vi "Write Binary Config.vi"(4 "Include Class Name":bool, 6 "byte order (0:big-endian, network order)":T1(ring), 8 "error in (no error)":errorcluster, 11 "Const_WFM in":refnum<class "Const_WFM_1D.lvclass">) -> (0 "error out":errorcluster, 2 "Binary":string, 3 "Const_WFM out":refnum<class "Const_WFM_1D.lvclass">)   [LabVIEW 2021, in "Const_WFM_1D.lvclass"]
uses:
  Const_WFM_1D.lvclass
  Const_WFM_1D.lvclass/Const_WFM_1D.ctl
  Abs_Types/Waveform 1D/Abs_Waveform 1D.lvclass
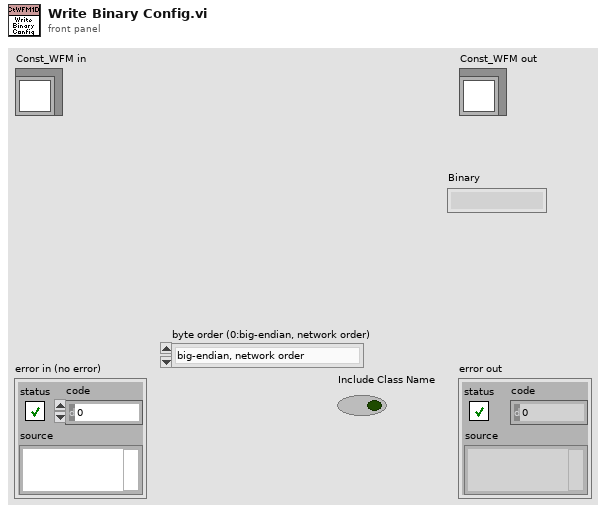
[diagram p1: front panel]
types:
  T1 = enum16{"big-endian, network order", "native, host order", "little-endian"}
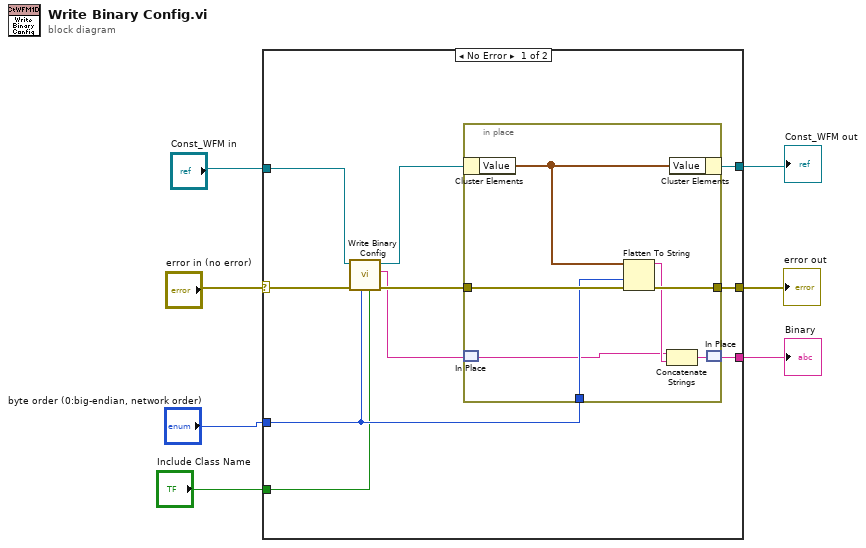
[diagram p0: block diagram]
diagram:
  n1 = case shown="No Error" "error in (no error)" {
    selector: "error in (no error)" -> [w17 w25]
    tunnel: [w13 w25] -> w7
    tunnel: [w8 w26] -> w5
    tunnel: "byte order (0:big-endian, network order)" -> [w14 _]
    tunnel: "Const_WFM in" -> [w16 w26]
    tunnel: [w11 _] -> w4
    tunnel: "Include Class Name" -> [w10 _]
    frame No Error {
      n2 = call-parent "Write Binary Config.vi"("Include Class Name"=w10, "byte order (0:big-endian, network order)"=w14, "error in (no error)"=w17, "Abs_Type in"=w16) -> ("error out"=w15:errorcluster, "Binary"=w12:string, "Abs_Type out"=w9:refnum<class "Const_WFM_1D.lvclass">)  [unwired: 5 in]
      n3 = in-place {
        in-place-border: w15 -> [w24]
        in-place-border: w14 -> [w23]
        in-place-border: [w22] -> w13
        n4 = in-place-cluster #1(w9) -> ("Value"=w18:waveform(dbl)[])
        n5 = in-place-match #2(w12) -> (w20:string)
        n6 = Flatten To String(anything=w18, byte order (0:big-endian, network order)=w23, error in (no error)=w24) -> (data string=w21:string, error out=w22:errorcluster)  [unwired: 1 in, 1 out]
        n7 = Concatenate Strings(w20, w21) -> (w19:string)
        n8 = in-place-cluster #1("Value"=w18) -> (w8:refnum<class "Const_WFM_1D.lvclass">)
        n9 = in-place-match #2(w19) -> (w11:string)
      }
    }
    frame Error {
    }
  }
  "error out" <- w7
  "Const_WFM out" <- w5
  "Binary" <- w4
